vi "Posicionador_VF_2.vi"() -> ()   [LabVIEW 2015]
uses:
  <vilib>/Instr/_visa.llb/VISA Configure Serial Port (Instr).vi
panel:
  out "Caracterización Terminada":bool
  in  "Puerto Serial del Gaussmetro":refnum<visa-resource-name>="COM5"
  in  "Ruta de archivo de medición":path=path "C:/Users/PIV/Desktop/Enrico/prueba1.txt"
  in  "Dato de entrada para\nobtención de flujo magnético 2":string=":MEASure:FLUX?\n"
  out "Medición de campo magnético \nen Teslas [T]":string
  out "?":string="mm"
  out "?":string="mm"
  in  "Listo Y":bool
  in  "Listo X":bool
  in  "Abajo":bool
  in  "Arriba":bool
  in  "Derecha":bool
  in  "Izquierda":bool
  out "Posiciòn en eje X":i32
  out "Posiciòn en eje Y":i32
  in  "Longitud del imán":i32
  in  "Altura del imán":i32
  in  "Puerto Serial de Arduino":refnum<visa-resource-name>="COM12"
  # "Manual de uso para sistema de monitoreo y control de lecturas de flujo magnético y desplazamiento de posicionador:\n\nPARA LA SECCIÓN DE IDE DE ARDUINO: El archivo denominado \"motor2.ino\" se encuentra en la carpeta denominada \"Caracterización\", en el subfolder \"motor2\". \n\n1.  Los pines para la conexión del driver del motor con el arduino están indicados en el archivo \"motor2.ino\" mediante las variables \"DirPin\", \"StepPin\", \"EnnablePin\" para el motor en X, y \"DirPin2\", \"StepPin2\", \"EnnablePin2\", para el motor en Y. El primer pin refiere a la Dirección; el segundo es el pin para mandarle el tren de pulsos y el tercero para habilitar el motor.\n2.  Para modificar el desplazamiento de 1mm de ambos motores, se deberá modificar el archivo \"motor2.ino\" en la sección después del loop denominada \"void stepMotor\" y \"void Stepmotor2, modificar la variable steps por la cantidad de desplazamiento deseado, tomando en cuenta que steps = 1000 = 1mm de desplazamiento.\n\nPARA LA SECCIÓN DEL EJECUTABLE: El archivo denominado \"Posicionador_VF.exe\" se encuentra en la carpeta \"Caracterización\".\n\n3.  En el apartado \"Puerto Serial de Arduino\" en la parte superior izquierda, indicar el puerto serial del Arduino. Para verificar en qué puerto se localiza, dirigirse al menú inicio y escribir \"Administrador de dispositivos\". Seguido de esto se darà click en la opciòn con el mismo nombre y, en la ventana que emerge, se buscarà el apartado \"Puertos COM y LPT\". El puerto del Arduino lleva por nombre inicial \"Arduino\".\n4.  Para seleccionar el puerto del Gaussmetro, dirigirse como en el paso anterior al Administrador de dispositivos y en el apartado Puerto COM y LPT buscar el nombre \"Prolific USB-to-Serial Comm Port\", y el nombre del puerto se especificará entre paréntesis. Este nombre de puerto se especificará en el apartado \"Puerto Serial del Gaussmetro\" ubicado debajo del apartado \"Puerto Serial de Arduino\". \n5.  Ingresar la longitud [en mm] del imán.\n6.  Ingresar el alto [en mm] del imán\n7.  Crear un archivo de texto .txt en la computadora (ubicación a elección) para guardar archivos \n8.  En el apartado \"Ruta de archivo de medición\" se deberá introducir la ubicación del archivo creado en el paso anterior. De esta manera, se introducirán las mediciones en este archivo.\n9.  En el apartado \"Dato de entrada para obtención de campo magnético\" se encuentra escrito el comando paara que el Gaussmetro arroje la medición de campo magnético.\n10.  Colocar el imán a caracterizar de forma que la probeta se encuentre del lado superior izquierdo de este. Esto debido a que el movimiento horizontal es hacia la derecha, y el movimiento vertical es hacia abajo.\n11.  Iniciar programa mediante la flecha (con dirección a la derecha) blanca en la parte superior izquierda del panel frontal o Ctrl+R.\n12. Verificar Conexión entre el Arduino y el posicionador. Esto se realiza observando un foco led color naranja en el motor (esto indica que la comunicación serial fue exitosa).\n13.  En caso de estar apagada la luz led naranja del motor, se deberá reiniciar el programa. Esto se consigue oprimiendo el boton \"Listo X\". Al hacer esto, se encenderá el led naranja, y de esta manera se procede a apagar el programa mediante el botón rojo de la parte superior izquierda del panel frontal. Después de realizar esta acciòn, volver a ejecutar el progama oprimiendo la flecha blanca a la izquierda del botón rojo o CTRL+R\n14.  Se deberá iniciar colocando la posición inicial en X (Derecha e Izquierda). Una vez finalizada la posición inicial en X, oprimir el botón \"Listo X\". Al finalizar, deberá parpadear una vez el foco led naranja y se volverá a encender.\n15.  Seguido, se colocará la  posición inicial en Y (Arriba y Abajo). Una vez finalizada la posición inicial en Y, oprimir el botón \"Listo Y\". Al finalizar, deberá parpadear una vez el foco led naranja y se volverá a encender.\n16.  Se comenzará la caracterización deseada.\n\n\nCreado por:\nSebastian A. Reyes Romero\nContacto: rerosa@ier.unam.mx"
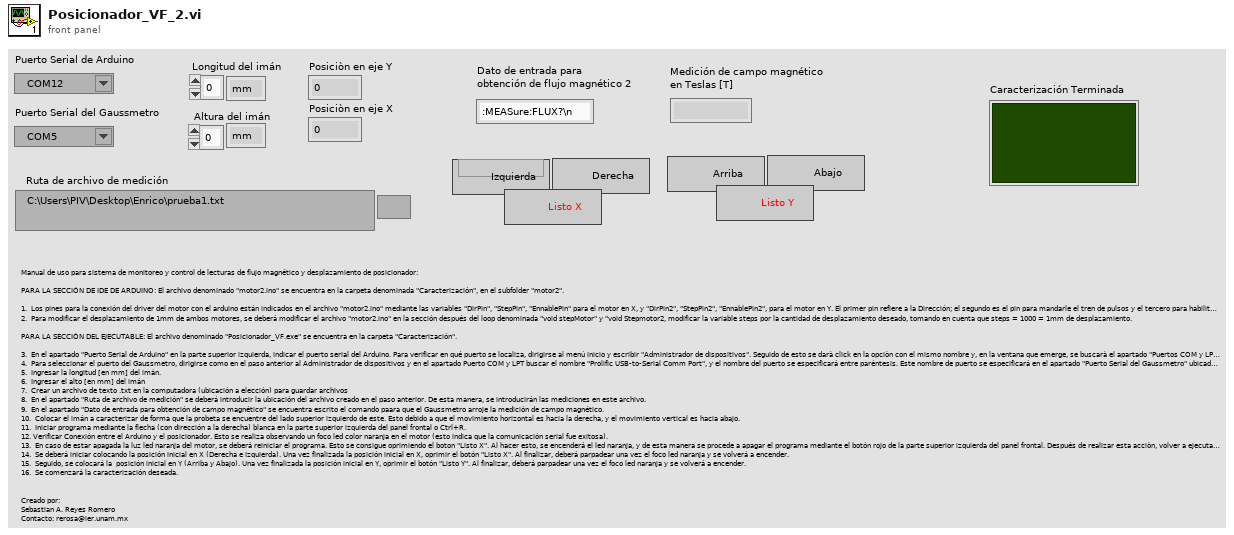
[diagram p1: front panel]
types:
  T1 = enum16{"open", "open or create", "create or replace", "create", "open (read only)"}
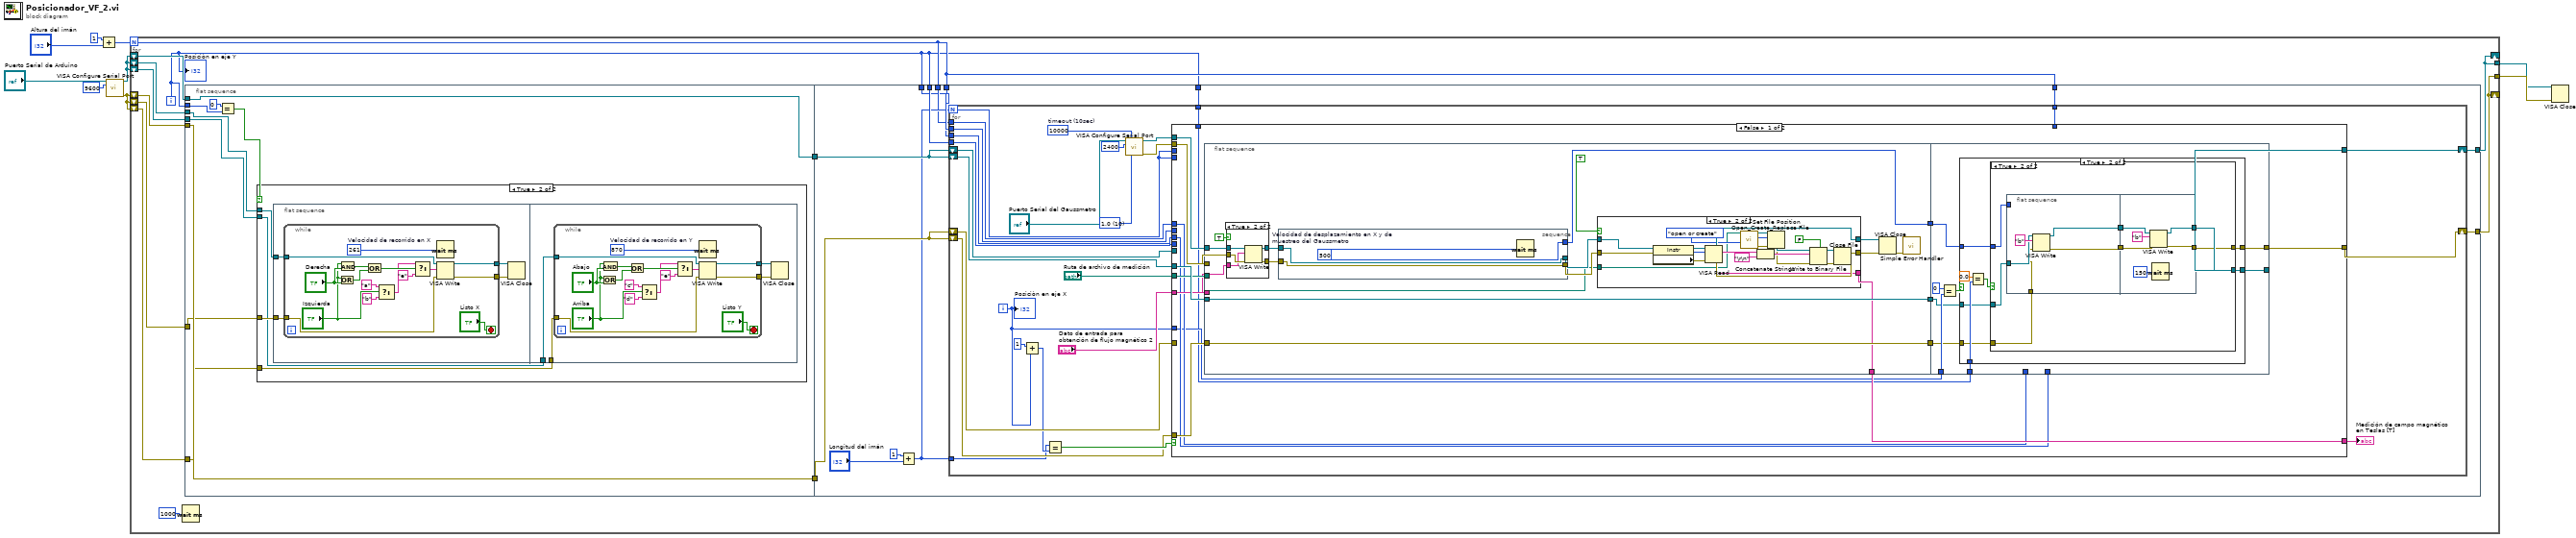
[diagram p0: block diagram]
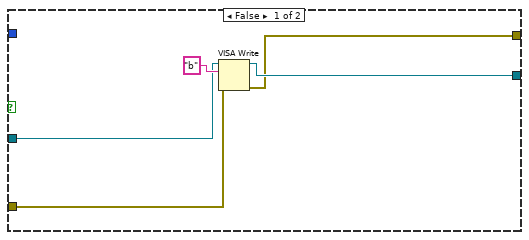
[diagram p5: hidden frame]
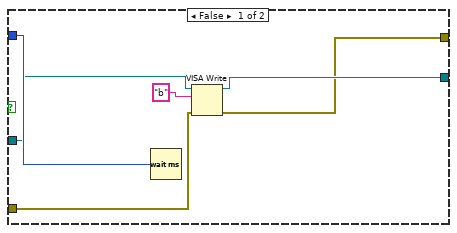
[diagram p6: hidden frame]
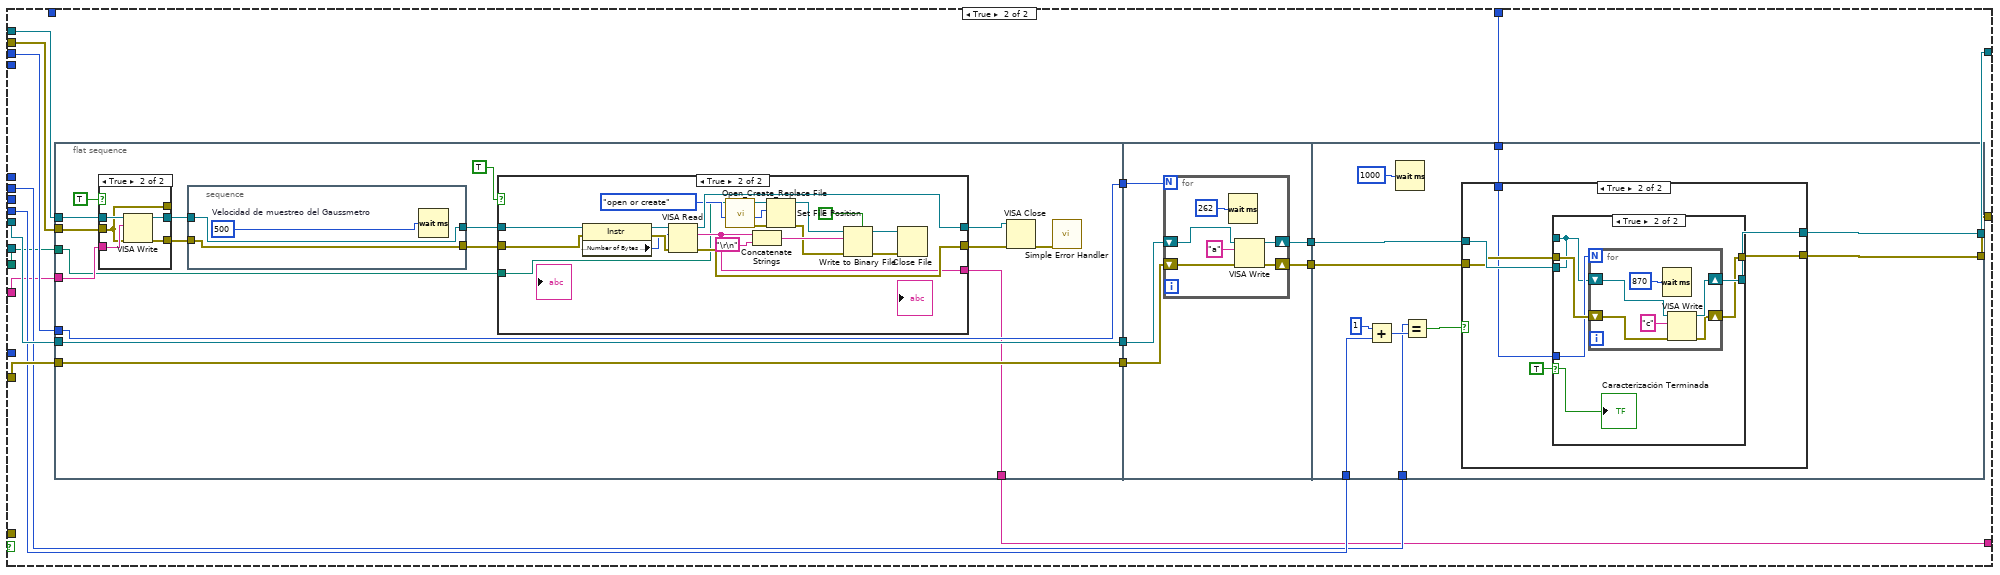
[diagram p7: hidden frame]
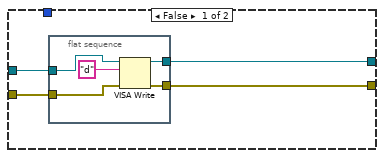
[diagram p10: hidden frame]
diagram:
  n1 = Add(x=1, y="Altura del imán") -> (x+y=w5:i32)
  n2 = call-poly "VISA Configure Serial Port"("VISA resource name"="Puerto Serial de Arduino", "baud rate (9600)"=u32 9600) -> ("VISA resource name out"=w3:refnum<visa-resource-name>, "error out"=w4:errorcluster)  [unwired: 12 in]
  n3 = for {
    N: w5 -> [w11]
    shift-right: [w12] -> _
    shift-right: [w13] -> _
    shift-left: w4 -> [w22]
    shift-left: w3 -> [w18]
    shift-left: w4 -> [w17]
    shift-left: w4 -> [w16]
    shift-left: w3 -> [w14]
    shift-left: w3 -> [w15]
    tunnel: [w13] -> w2
    tunnel: [w12] -> w1
    i -> [w10]
    n4 = Wait (ms)(milliseconds to wait=u32 1000) -> ()  [unwired: 1 out]
    n5 = flat-sequence {
      tunnel: w22 -> [w31]
      tunnel: [w28] -> w20
      tunnel: [w31] -> w19
      tunnel: w18 -> [w27]
      tunnel: w17 -> [w30]
      tunnel: w16 -> [w29]
      tunnel: w15 -> [w28]
      tunnel: w14 -> [w26]
      tunnel: w10 -> [w25]
      tunnel: [w87] -> w13
      tunnel: [w88] -> w12
      tunnel: w10 -> [w84]
      tunnel: w11 -> [w83]
      tunnel: w20 -> [w86]
      tunnel: w19 -> [w85]
      tunnel: w11 -> [w79]
      tunnel: w10 -> [w78]
      tunnel: w11 -> [w77]
      tunnel: w10 -> [w76]
      frame #0 {
        n6 = Equal?(x=0, y=w25) -> (x = y?=w23:bool)
        n7 = case shown="True" w23 {
          tunnel: w30 -> [_ w35]
          tunnel: w29 -> [_ w34]
          tunnel: w27 -> [_ w33]
          tunnel: w26 -> [_ w32]
          frame False {
          }
          frame True {
            n8 = flat-sequence {
              tunnel: w32 -> [w39]
              tunnel: w35 -> [w38]
              tunnel: w33 -> [w59]
              tunnel: w34 -> [w58]
              frame #0 {
                n9 = while {
                  tunnel: w39 -> [w46]
                  tunnel: w38 -> [w45]
                  tunnel: [w41] -> w37
                  tunnel: [w40] -> w36
                  stop <- "Listo X" stop-if-true
                  w42 = u32 261  # Velocidad de recorrido en X
                  n10 = Or(x="Izquierda", y="Derecha") -> (x .or. y?=w52:bool)
                  n11 = And(x="Izquierda", y="Derecha") -> (x .and. y?=w54:bool)
                  n12 = Or(x=w54, y=w52) -> (x .or. y?=w51:bool)
                  n13 = Select(t="a", s="Izquierda", f="b") -> (s? t:f=w44:string)
                  n14 = Select(t=w44, s=w51, f="e") -> (s? t:f=w47:string)
                  n15 = Wait (ms)(milliseconds to wait=w42) -> ()  [unwired: 1 out]
                  n16 = VISA Write(VISA resource name=w46, write buffer=w47, error in (no error)=w45) -> (VISA resource name out=w40:refnum<visa-resource-name>, error out=w41:errorcluster)  [unwired: 1 out]
                }
                n17 = VISA Close(VISA resource name=w36, error in (no error)=w37) -> ()  [unwired: 1 out]
              }
              frame #1 {
                n18 = while {
                  tunnel: w59 -> [w66]
                  tunnel: w58 -> [w65]
                  tunnel: [w61] -> w57
                  tunnel: [w60] -> w56
                  stop <- "Listo Y" stop-if-true
                  w62 = u32 870  # Velocidad de recorrido en Y
                  n19 = Or(x="Arriba", y="Abajo") -> (x .or. y?=w73:bool)
                  n20 = And(x="Arriba", y="Abajo") -> (x .and. y?=w74:bool)
                  n21 = Or(x=w74, y=w73) -> (x .or. y?=w72:bool)
                  n22 = Select(t="c", s="Arriba", f="d") -> (s? t:f=w63:string)
                  n23 = Select(t=w63, s=w72, f="e") -> (s? t:f=w67:string)
                  n24 = Wait (ms)(milliseconds to wait=w62) -> ()  [unwired: 1 out]
                  n25 = VISA Write(VISA resource name=w66, write buffer=w67, error in (no error)=w65) -> (VISA resource name out=w60:refnum<visa-resource-name>, error out=w61:errorcluster)  [unwired: 1 out]
                }
                n26 = VISA Close(VISA resource name=w56, error in (no error)=w57) -> ()  [unwired: 1 out]
              }
            }
          }
        }
      }
      frame #1 {
        n27 = Add(x=1, y="Longitud del imán") -> (x+y=w80:i32)
        n28 = for {
          N: w80 -> [w109]
          shift-right: [w112] -> w88
          shift-left: w86 -> [w114]
          shift-right: [w111] -> w87
          shift-left: w85 -> [w113]
          shift-left: w86 -> [w110]
          shift-left: w85 -> [w108]
          tunnel: w80 -> [w105]
          tunnel: w84 -> [w104]
          tunnel: w83 -> [w103]
          tunnel: w79 -> [w93]
          tunnel: w78 -> [w92]
          tunnel: w77 -> [w91]
          tunnel: w76 -> [w89]
          i -> [w90]
          w96 = u16 10 items=["1.0"=10, "1.5"=15, "2.0"=20] ("stop bits (10: 1 bit)")
          w99 = u32 10000  # timeout (10sec)
          n29 = Add(x=1, y=w90) -> (x+y=w106:i32)
          n30 = Equal?(x=w105, y=w106) -> (x = y?=w115:bool)
          n31 = call-poly "VISA Configure Serial Port"("VISA resource name"="Puerto Serial del Gaussmetro", "timeout (10sec)"=w99, "baud rate (9600)"=u32 2400, "stop bits (10: 1 bit)"=w96) -> ("VISA resource name out"=w95:refnum<visa-resource-name>, "error out"=w94:errorcluster)  [unwired: 5 in, 5 out]
          n32 = case shown="False" w115 {
            tunnel: w114 -> [_ w244]
            tunnel: w113 -> [_ w243]
            tunnel: [w129 w242] -> w112
            tunnel: [w128 w241] -> w111
            tunnel: w109 -> [_ w240]
            tunnel: w110 -> [w131 _]
            tunnel: w108 -> [w130 _]
            tunnel: w109 -> [_ _]
            tunnel: w104 -> [_ w237]
            tunnel: w103 -> [_ w236]
            tunnel: [w124 w232] -> w102
            tunnel: "Dato de entrada para\nobtención de flujo magnético 2" -> [w123 w231]
            tunnel: "Ruta de archivo de medición" -> [w122 w230]
            tunnel: w95 -> [w121 w229]
            tunnel: w94 -> [w120 w228]
            tunnel: w93 -> [w119 _]
            tunnel: w92 -> [w118 _]
            tunnel: w91 -> [_ w227]
            tunnel: w90 -> [w117 _]
            tunnel: w89 -> [w116 _]
            frame False {
              n33 = flat-sequence {
                tunnel: w130 -> [w147]
                tunnel: w131 -> [w148]
                tunnel: [w148] -> w127
                tunnel: [w147] -> w126
                tunnel: [w137] -> w125
                tunnel: [w136] -> w124
                tunnel: w123 -> [w135]
                tunnel: w122 -> [w134]
                tunnel: w121 -> [w133]
                tunnel: w120 -> [w132]
                tunnel: [w182] -> w128
                tunnel: [w183] -> w129
                tunnel: w119 -> [_]
                tunnel: w118 -> [_]
                tunnel: w125 -> [w181]
                tunnel: w126 -> [w184]
                tunnel: w127 -> [w185]
                tunnel: w117 -> [w189]
                tunnel: w116 -> [w186]
                frame #0 {
                  n34 = case shown="True" TRUE ("write") {
                    tunnel: [w153 w158] -> w141
                    tunnel: w133 -> [w152 w157]
                    tunnel: w132 -> [w153 w156]
                    tunnel: [w152 w155] -> w139
                    tunnel: w135 -> [_ w154]
                    frame False {
                    }
                    frame True {
                      n35 = VISA Write(VISA resource name=w157, write buffer=w154, error in (no error)=w156) -> (VISA resource name out=w155:refnum<visa-resource-name>, error out=w158:errorcluster)  [unwired: 1 out]
                    }
                  }
                  n36 = stacked-sequence {
                    tunnel: w141 -> [w151]
                    tunnel: [w151] -> w140
                    tunnel: w139 -> [w150]
                    tunnel: [w150] -> w138
                    tunnel: [w149] -> w137
                    frame #0 {
                      w149 = u32 500  # Velocidad de desplazamiento en X y de muestreo del Gaussmetro
                      n37 = Wait (ms)(milliseconds to wait=w149) -> ()  [unwired: 1 out]
                    }
                  }
                  n38 = case shown="True" TRUE ("read") {
                    tunnel: w140 -> [w160 w177]
                    tunnel: [w160 w174] -> w145
                    tunnel: [w159 w180] -> w144
                    tunnel: w138 -> [w159 w179]
                    tunnel: [_ w162] -> w136
                    tunnel: w134 -> [_ w161]
                    frame False {
                    }
                    frame True {
                      n39 = property class="Instr"(reference=w179, error in=w177) -> (reference out=w178:refnum<visa-resource-name>, error out=w176:errorcluster, "Serial Settings:Number of Bytes at Serial Port"=w175:u32)
                      n40 = VISA Read(VISA resource name=w178, byte count=w175, error in (no error)=w176) -> (VISA resource name out=w180:refnum<visa-resource-name>, read buffer=w162:string, error out=w174:errorcluster)  [unwired: 1 out]
                      n41 = call <vilib>:"Open_Create_Replace File.vi"("function (open:0)"=T1."open or create", "file path"=w161) -> ("error out"=w172:errorcluster, "file size (bytes)"=w170:i32, "refnum"=w171:refnum<file>)  [unwired: 6 in, 1 out]
                      n42 = Concatenate Strings(w162, "\r\n") -> (w166:string)
                      n43 = Set File Position(offset (in bytes) (0)=w170, refnum=w171, error in=w172) -> (refnum out=w165:refnum<file>, error out=w164:errorcluster)  [unwired: 1 in]
                      n44 = Write to Binary File(file (use dialog)=w165, data=w166, error in=w164, 5:FALSE ("prepend array or string size? (T)")) -> (refnum out=w168:refnum<file>, error out=w169:errorcluster)  [unwired: 2 in, 1 out]
                      n45 = Close File(refnum=w168, error in=w169) -> ()  [unwired: 2 out]
                    }
                  }
                  n46 = VISA Close(VISA resource name=w144, error in (no error)=w145) -> (error out=w143:errorcluster)
                  n47 = call <vilib>:"Simple Error Handler.vi"("error in (no error)"=w143) -> ()  [unwired: 1 in, 8 out]
                }
                frame #1 {
                  n48 = Equal?(x=0, y=w189) -> (x = y?=w188:bool)
                  n49 = case shown="True" w188 {
                    tunnel: w186 -> [_ w200]
                    tunnel: w185 -> [w193 w199]
                    tunnel: w184 -> [w192 w198]
                    tunnel: [w191 w197] -> w183
                    tunnel: [w190 w196] -> w182
                    tunnel: w181 -> [_ w195]
                    frame False {
                      n50 = VISA Write(VISA resource name=w193, write buffer="b", error in (no error)=w192) -> (VISA resource name out=w191:refnum<visa-resource-name>, error out=w190:errorcluster)  [unwired: 1 out]
                    }
                    frame True {
                      n51 = Equal?(x=0.0, y=w200) -> (x = y?=w202:bool)
                      n52 = case shown="True" w202 {
                        tunnel: w199 -> [w206 w215]
                        tunnel: w198 -> [w205 w214]
                        tunnel: [w204 w213] -> w197
                        tunnel: [w203 w212] -> w196
                        tunnel: w195 -> [w207 w209]
                        frame False {
                          n53 = Wait (ms)(milliseconds to wait=w207) -> ()  [unwired: 1 out]
                          n54 = VISA Write(VISA resource name=w206, write buffer="b", error in (no error)=w205) -> (VISA resource name out=w204:refnum<visa-resource-name>, error out=w203:errorcluster)  [unwired: 1 out]
                        }
                        frame True {
                          n55 = flat-sequence {
                            tunnel: w215 -> [w219]
                            tunnel: w214 -> [w218]
                            tunnel: [w217] -> w211
                            tunnel: [w216] -> w210
                            tunnel: w209 -> [_]
                            tunnel: [w222] -> w212
                            tunnel: [w224] -> w213
                            tunnel: w211 -> [w225]
                            tunnel: w210 -> [w223]
                            frame #0 {
                              n56 = VISA Write(VISA resource name=w219, write buffer="b", error in (no error)=w218) -> (VISA resource name out=w217:refnum<visa-resource-name>, error out=w216:errorcluster)  [unwired: 1 out]
                            }
                            frame #1 {
                              n57 = VISA Write(VISA resource name=w225, write buffer="b", error in (no error)=w223) -> (VISA resource name out=w224:refnum<visa-resource-name>, error out=w222:errorcluster)  [unwired: 1 out]
                              n58 = Wait (ms)(milliseconds to wait=u32 150) -> ()  [unwired: 1 out]
                            }
                          }
                        }
                      }
                    }
                  }
                }
              }
            }
            frame True {
              n59 = flat-sequence {
                tunnel: w240 -> [w259]
                tunnel: w243 -> [w260]
                tunnel: w244 -> [w261]
                tunnel: [w261] -> w235
                tunnel: [w260] -> w234
                tunnel: [w259] -> w233
                tunnel: [w249] -> w232
                tunnel: w231 -> [w248]
                tunnel: w230 -> [w247]
                tunnel: w229 -> [w246]
                tunnel: w228 -> [w245]
                tunnel: [w296] -> w239
                tunnel: [w295] -> w238
                tunnel: w235 -> [w298]
                tunnel: w234 -> [w297]
                tunnel: w233 -> [w294]
                tunnel: [w314] -> w241
                tunnel: [w315] -> w242
                tunnel: w236 -> [w308]
                tunnel: w237 -> [w311]
                tunnel: w238 -> [w312]
                tunnel: w239 -> [w313]
                tunnel: w227 -> [w305]
                frame #0 {
                  n60 = case shown="True" TRUE ("write 2") {
                    tunnel: [w265 w271] -> w253
                    tunnel: w246 -> [w266 w270]
                    tunnel: [w265 w267] -> _
                    tunnel: [w266 w269] -> w251
                    tunnel: w248 -> [_ w268]
                    tunnel: w245 -> [w265 w267]
                    frame False {
                    }
                    frame True {
                      n61 = VISA Write(VISA resource name=w270, write buffer=w268, error in (no error)=w267) -> (VISA resource name out=w269:refnum<visa-resource-name>, error out=w271:errorcluster)  [unwired: 1 out]
                    }
                  }
                  n62 = stacked-sequence {
                    tunnel: w253 -> [w264]
                    tunnel: [w264] -> w252
                    tunnel: w251 -> [w263]
                    tunnel: [w263] -> w250
                    frame #0 {
                      w262 = u32 500  # Velocidad de muestreo del Gaussmetro
                      n63 = Wait (ms)(milliseconds to wait=w262) -> ()  [unwired: 1 out]
                    }
                  }
                  n64 = case shown="True" TRUE ("read 2") {
                    tunnel: w252 -> [w273 w290]
                    tunnel: [w273 w287] -> w257
                    tunnel: [w272 w293] -> w256
                    tunnel: w250 -> [w272 w292]
                    tunnel: [_ w275] -> w249
                    tunnel: w247 -> [_ w274]
                    frame False {
                    }
                    frame True {
                      n65 = property class="Instr"(reference=w292, error in=w290) -> (reference out=w291:refnum<visa-resource-name>, error out=w289:errorcluster, "Serial Settings:Number of Bytes at Serial Port"=w288:u32)
                      n66 = VISA Read(VISA resource name=w291, byte count=w288, error in (no error)=w289) -> (VISA resource name out=w293:refnum<visa-resource-name>, read buffer=w275:string, error out=w287:errorcluster)  [unwired: 1 out]
                      n67 = call <vilib>:"Open_Create_Replace File.vi"("function (open:0)"=T1."open or create", "file path"=w274) -> ("error out"=w285:errorcluster, "file size (bytes)"=w283:i32, "refnum"=w284:refnum<file>)  [unwired: 6 in, 1 out]
                      n68 = Concatenate Strings(w275, "\r\n") -> (w279:string)
                      n69 = Set File Position(offset (in bytes) (0)=w283, refnum=w284, error in=w285) -> (refnum out=w278:refnum<file>, error out=w277:errorcluster)  [unwired: 1 in]
                      n70 = Write to Binary File(file (use dialog)=w278, data=w279, error in=w277, 5:FALSE ("prepend array or string size? (T)")) -> (refnum out=w281:refnum<file>, error out=w282:errorcluster)  [unwired: 2 in, 1 out]
                      n71 = Close File(refnum=w281, error in=w282) -> ()  [unwired: 2 out]
                    }
                  }
                  n72 = VISA Close(VISA resource name=w256, error in (no error)=w257) -> (error out=w255:errorcluster)
                  n73 = call <vilib>:"Simple Error Handler.vi"("error in (no error)"=w255) -> ()  [unwired: 1 in, 8 out]
                }
                frame #1 {
                  n74 = for {
                    N: w294 -> [_]
                    shift-right: [w302] -> w296
                    shift-left: w298 -> [w304]
                    shift-right: [w301] -> w295
                    shift-left: w297 -> [w303]
                    n75 = Wait (ms)(milliseconds to wait=u32 262) -> ()  [unwired: 1 out]
                    n76 = VISA Write(VISA resource name=w304, write buffer="a", error in (no error)=w303) -> (VISA resource name out=w302:refnum<visa-resource-name>, error out=w301:errorcluster)  [unwired: 1 out]
                  }
                }
                frame #2 {
                  n77 = Add(x=1, y=w311) -> (x+y=w309:i32)
                  n78 = Wait (ms)(milliseconds to wait=u32 1000) -> ()  [unwired: 1 out]
                  n79 = Equal?(x=w308, y=w309) -> (x = y?=w307:bool)
                  n80 = case shown="True" w307 {
                    tunnel: w313 -> [w319 w330]
                    tunnel: [w318 w328] -> w315
                    tunnel: w312 -> [w317 w329]
                    tunnel: [w316 w327] -> w314
                    tunnel: w305 -> [_ w326]
                    frame False {
                      n81 = flat-sequence {
                        tunnel: [w323] -> w316
                        tunnel: [w324] -> w318
                        tunnel: w317 -> [w321]
                        tunnel: w319 -> [w322]
                        frame #0 {
                          n82 = VISA Write(VISA resource name=w322, write buffer="d", error in (no error)=w321) -> (VISA resource name out=w324:refnum<visa-resource-name>, error out=w323:errorcluster)  [unwired: 1 out]
                        }
                      }
                    }
                    frame True {
                      n83 = case shown="True" TRUE {
                        selector: TRUE -> [_ w333]
                        tunnel: [w331 w334] -> _
                        tunnel: w329 -> [w332 w338]
                        tunnel: [w331 w337] -> w328
                        tunnel: [w332 w336] -> w327
                        tunnel: w326 -> [_ w335]
                        tunnel: w330 -> [w331 w334]
                        frame False {
                        }
                        frame True {
                          n84 = for {
                            N: w335 -> [_]
                            shift-right: [w342] -> w337
                            shift-left: w334 -> [w344]
                            shift-right: [w341] -> w336
                            shift-left: w338 -> [w343]
                            n85 = Wait (ms)(milliseconds to wait=u32 870) -> ()  [unwired: 1 out]
                            n86 = VISA Write(VISA resource name=w344, write buffer="c", error in (no error)=w343) -> (VISA resource name out=w342:refnum<visa-resource-name>, error out=w341:errorcluster)  [unwired: 1 out]
                          }
                          "Caracterización Terminada" <- w333
                        }
                      }
                    }
                  }
                }
              }
            }
          }
          "Medición de campo magnético \nen Teslas [T]" <- w102
          "Posiciòn en eje X" <- w90
        }
      }
    }
    "Posiciòn en eje Y" <- w10
  }
  n87 = VISA Close(VISA resource name=w1, error in (no error)=w2) -> ()  [unwired: 1 out]
